vi "Drive Control.vi"(6 "GyroDevRef":T2={"DevStatus"={"status"=FALSE, "code"=0, "source"=""}, "Analog Module"=enum."Analog Module 1", "Analog Channel"=enum."Invalid", "Offset"=0.0, "Gain (VoltsPerDegree/Second)"=0.0}, 8 "Buttons":T1, 9 "rotation":dbl, 10 "y":dbl, 11 "x":dbl) -> (1 "Rotation":dbl, 2 "Direction":dbl, 3 "Speed":dbl)   [LabVIEW 2013]
uses:
  <vilib>/Rock Robotics/WPI/Gyro/WPI_GyroDevRef.ctl
  <vilib>/Rock Robotics/SystemInterfaces/Typedef/FPGA_TypedefAnalogModule.ctl
  <vilib>/Rock Robotics/SystemInterfaces/AI/FPGA_AIChannel.ctl
  Utils/XBox Buttons.ctl
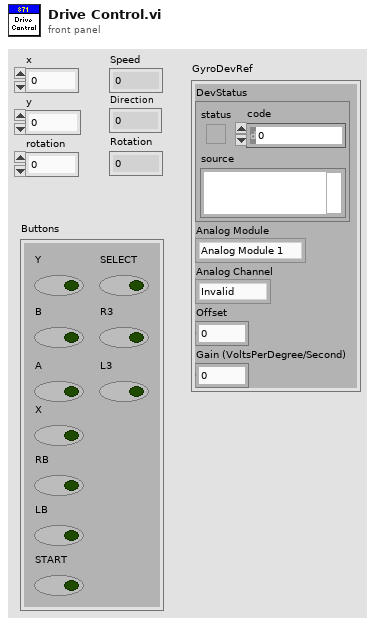
[diagram p1: front panel]
types:
  T1 = typedef "XBox Buttons.ctl" = cluster{"Y":bool, "B":bool, "A":bool, "X":bool, "RB":bool, "LB":bool, "START":bool, "SELECT":bool, "R3":bool, "L3":bool}
  T2 = typedef "WPI_GyroDevRef.ctl" = cluster{"DevStatus":errorcluster, "Analog Module":T3, "Analog Channel":T4, "Offset":dbl, "Gain (VoltsPerDegree/Second)":dbl}
  T3 = typedef "FPGA_TypedefAnalogModule.ctl" = enum16{"Analog Module 1", "Analog Module 2"}
  T4 = typedef "FPGA_AIChannel.ctl" = enum8{"AI 1", "AI 2", "AI 3", "AI 4", "AI 5", "AI 6", "AI 7", "AI 8", "Invalid"}
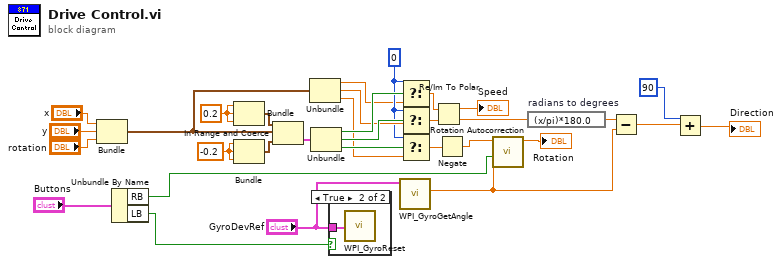
[diagram p0: block diagram]
diagram:
  w18 = 0
  w27 = -0.2
  w29 = 0.2
  n1 = Bundle("x"="x", "y"="y", "rotation"="rotation") -> (w12:cluster{"x":dbl, "y":dbl, "rotation":dbl})  [unwired: 1 in]
  n2 = Unbundle By Name("Buttons") -> ("RB"=w3:bool, "LB"=w5:bool)
  n3 = Bundle(w29, w29, w29) -> (w28:cluster{dbl, dbl, dbl})  [unwired: 1 in]
  n4 = Bundle(w27, w27, w27) -> (w26:cluster{dbl, dbl, dbl})  [unwired: 1 in]
  n5 = In Range and Coerce(upper limit=w28, x=w12, lower limit=w26) -> (In Range?=w24:cluster{"x":bool, "y":bool, "rotation":bool})  [unwired: 1 out]
  n6 = Unbundle(w12) -> ("x"=w11:dbl, "y"=w20:dbl, "rotation"=w19:dbl)
  n7 = Unbundle(w24) -> ("x"=w21:bool, "y"=w22:bool, "rotation"=w23:bool)
  n8 = case shown="True" w5 {
    tunnel: "GyroDevRef" -> [_ w33]
    frame False {
    }
    frame True {
      n9 = call <vilib>:"WPI_GyroReset.vi"("GyroDevRef"=w33) -> ()  [unwired: 9 in, 2 out]
    }
  }
  n10 = call <vilib>:"WPI_GyroGetAngle.vi"("GyroDevRef"="GyroDevRef") -> ("Angle"=w2:dbl)  [unwired: 7 in, 3 out]
  n11 = Select(t=w18, s=w21, f=w11) -> (s? t:f=w17:dbl)
  n12 = Select(t=w18, s=w22, f=w20) -> (s? t:f=w16:dbl)
  n13 = Select(t=w18, s=w23, f=w19) -> (s? t:f=w7:dbl)
  n14 = Re/Im To Polar(2:w16, 3:w17) -> (0:w14:dbl, 1:→"Speed":dbl)
  n15 = Negate(x=w7) -> (-x=w4:dbl)
  n16 = call "Rotation Autocorrection.vi"("Gyro"=w2, "Enable\nAutocorrect"=w3, "Rotation"=w4) -> ("Rotation corrected"=→"Rotation":dbl)  [unwired: 8 in]
  n17 = expression code="(x/pi)*180.0" "radians to degrees"(w14) -> (w13:dbl)
  n18 = Subtract(x=w13, y=w2) -> (x-y=w9:dbl)
  n19 = Add(x=90, y=w9) -> (x+y=→"Direction":dbl)
